vi "Filter Dead End Pixels (SubVI).vi"(0 "Data In":u8, 3 "In Valid?":bool) -> (14 "Data Out":u8, 18 "Out Valid?":bool)   [LabVIEW 2015]
doc: "Filters input image and remove objects that are smaller than 128 x 128 pixels in size."
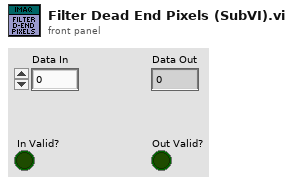
[diagram p1: front panel]
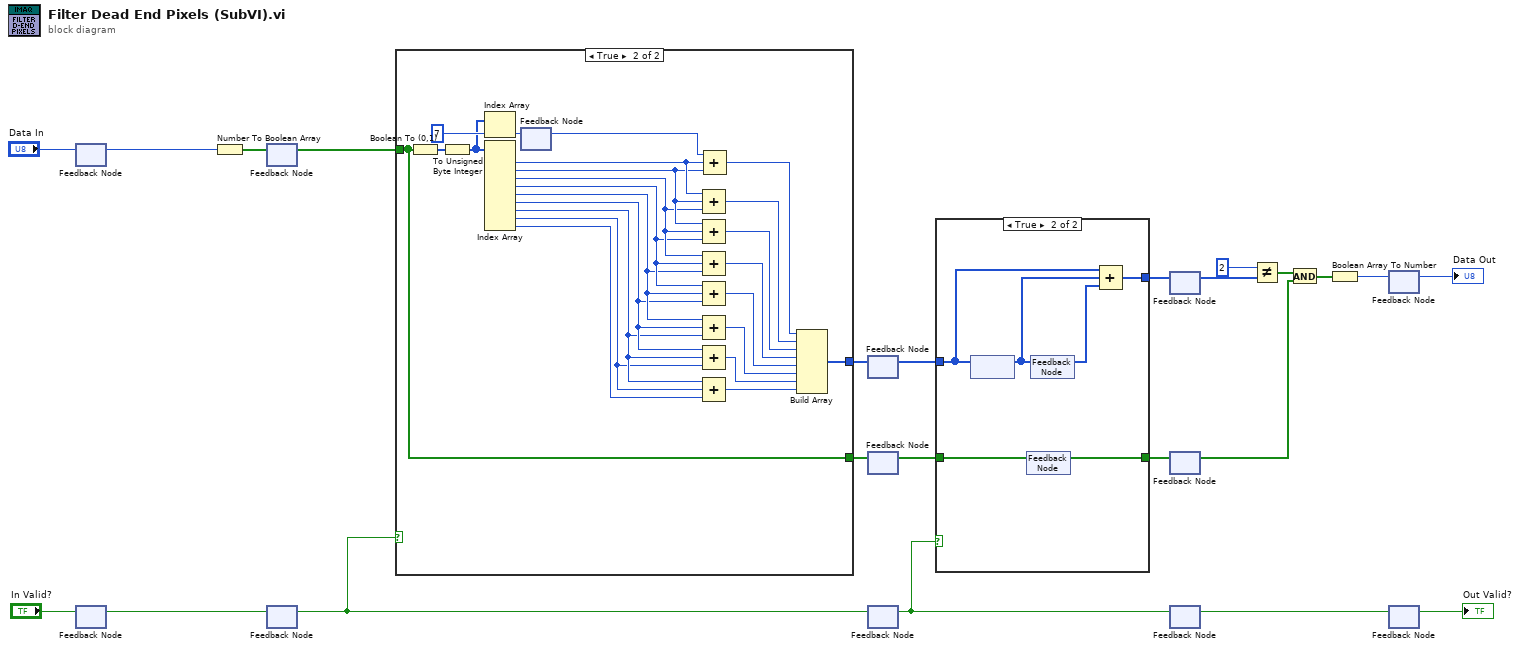
[diagram p0: block diagram]
diagram:
  n1 = feedback-in #1("Data In") -> ()
  n2 = feedback #1() -> (w8:u8)  [unwired: 1 in]
  n3 = feedback-in #2("In Valid?") -> ()
  n4 = feedback #2() -> (w12:bool)  [unwired: 1 in]
  n5 = Number To Boolean Array(number=w8) -> (Boolean array=w16:bool[])
  n6 = feedback-in #3(w16) -> ()
  n7 = feedback #3() -> (w21:bool[])  [unwired: 1 in]
  n8 = feedback-in #4(w12) -> ()
  n9 = feedback #4() -> (w11:bool)  [unwired: 1 in]
  n10 = case shown="True" w11 {
    tunnel: [_ w31] -> w22
    tunnel: w21 -> [_ w24]
    tunnel: [_ w24] -> w5
    frame False {
    }
    frame True {
      n11 = Boolean To (0,1)(Boolean=w24) -> (0, 1=w46:i16[])
      n12 = To Unsigned Byte Integer(number=w46) -> (unsigned 8bit integer=w43:u8[])
      n13 = Index Array(array=w43, index=7) -> (element=w42:u8)
      n14 = Index Array(array=w43) -> (element #1=w41:u8, element #2=w39:u8, element #3=w38:u8, element #4=w37:u8, element #5=w36:u8, element #6=w35:u8, element #7=w34:u8, element #8=w33:u8, element #9=w32:u8)  [unwired: 9 in]
      n15 = feedback-in #5(w42) -> ()
      n16 = feedback #5() -> (w45:u8)  [unwired: 1 in]
      n17 = Compound Arithmetic op=ADD(w41, w39, w38) -> (w40:u8)
      n18 = Compound Arithmetic op=ADD(w39, w38, w37) -> (w30:u8)
      n19 = Compound Arithmetic op=ADD(w38, w37, w36) -> (w29:u8)
      n20 = Compound Arithmetic op=ADD(w37, w36, w35) -> (w28:u8)
      n21 = Compound Arithmetic op=ADD(w36, w35, w34) -> (w27:u8)
      n22 = Compound Arithmetic op=ADD(w35, w34, w33) -> (w26:u8)
      n23 = Compound Arithmetic op=ADD(w34, w33, w32) -> (w25:u8)
      n24 = Compound Arithmetic op=ADD(w45, w41, w39) -> (w47:u8)
      n25 = Build Array(w47, w40, w30, w29, w28, w27, w26, w25) -> (w31:u8[])
    }
  }
  n26 = feedback-in #6(w22) -> ()
  n27 = feedback #6() -> (w18:u8[])  [unwired: 1 in]
  n28 = feedback-in #7(w5) -> ()
  n29 = feedback #7() -> (w4:bool[])  [unwired: 1 in]
  n30 = feedback-in #8(w11) -> ()
  n31 = feedback #8() -> (w10:bool)  [unwired: 1 in]
  n32 = case shown="True" w10 {
    tunnel: [_ w53] -> w20
    tunnel: w18 -> [_ w52]
    tunnel: [_ w48] -> w2
    tunnel: w4 -> [_ w49]
    frame False {
    }
    frame True {
      n33 = feedback #9() -> (w51:u8[])  [unwired: 1 in]
      n34 = feedback-in #9(w52) -> ()
      n35 = feedback-in #10(w49) -> ()
      n36 = feedback #10() -> (w48:bool[])  [unwired: 1 in]
      n37 = feedback-in #11(w51) -> ()
      n38 = feedback #11() -> (w50:u8[])  [unwired: 1 in]
      n39 = Compound Arithmetic op=ADD(w52, w51, w50) -> (w53:u8[])
    }
  }
  n40 = feedback-in #12(w20) -> ()
  n41 = feedback #12() -> (w23:u8[])  [unwired: 1 in]
  n42 = feedback-in #13(w2) -> ()
  n43 = feedback #13() -> (w1:bool[])  [unwired: 1 in]
  n44 = feedback-in #14(w10) -> ()
  n45 = feedback #14() -> (w9:bool)  [unwired: 1 in]
  n46 = Not Equal?(x=u8 2 ("number"), y=w23) -> (x != y?=w7:bool[])
  n47 = And(x=w7, y=w1) -> (x .and. y?=w3:bool[])
  n48 = Boolean Array To Number(Boolean array=w3) -> (number=w15:u8)
  n49 = feedback-in #15(w15) -> ()
  n50 = feedback #15() -> (→"Data Out":u8)  [unwired: 1 in]
  n51 = feedback-in #16(w9) -> ()
  n52 = feedback #16() -> (→"Out Valid?":bool)  [unwired: 1 in]
